vi "Copy FPGA SCTL.vi"(8 "error in (no error)":errorcluster, 11 "SCTL Name":string) -> (0 "error out":errorcluster)   [LabVIEW 2025, in "VI.lvclass"]
doc: "Copy a STCL from a template VI to be pasted into another VI."
uses:
  VI.lvclass
  VI.lvclass/VI.ctl
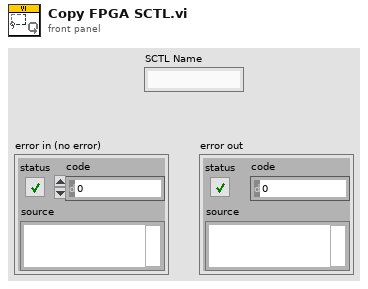
[diagram p1: front panel]
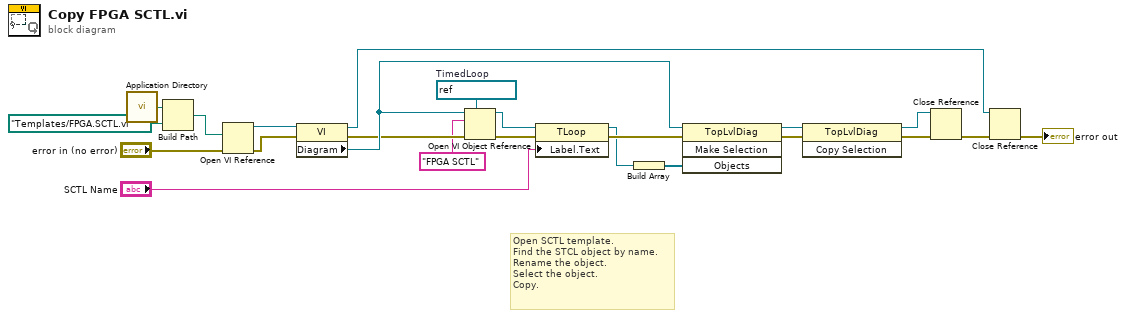
[diagram p0: block diagram]
diagram:
  w15 = refnum<vi> refnum  # TimedLoop
  # "Open SCTL template.\nFind the STCL object by name.\nRename the object.\nSelect the object.\nCopy."
  n1 = call <vilib>:"Application Directory.vi"() -> ("Application Directory"=w3:path)
  n2 = Build Path(base path=w3, name or relative path=path "Templates/FPGA.SCTL.vi" ("Application Directory")) -> (appended path=w1:path)
  n3 = Open VI Reference(vi path=w1, error in (no error)="error in (no error)") -> (vi reference=w9:refnum<vi>, error out=w13:errorcluster)  [unwired: 4 in]
  n4 = property class="VI"(reference=w9, error in=w13) -> (reference out=w20:refnum<vi>, error out=w17:errorcluster, "Diagram"=w18:refnum<vi>)
  n5 = Open VI Object Reference(7:w15, 8:w17, 10:"FPGA SCTL" ("name/order"), 11:w18) -> (0:w7:errorcluster, 3:w8:refnum<vi>)
  n6 = property class="TLoop"(reference=w8, error in=w7, "Label.Text"="SCTL Name") -> (reference out=w5:refnum<vi>, error out=w6:errorcluster)
  n7 = Build Array(w5) -> (w16:refnum<vi>[])
  n8 = invoke class="TopLvlDiag" method="Make Selection"(reference=w18, error in=w6, "Objects"=w16) -> (reference out=w10:refnum<vi>, error out=w11:errorcluster)  [unwired: 1 in, 2 out]
  n9 = invoke class="TopLvlDiag" method="Copy Selection"(reference=w10, error in=w11) -> (reference out=w22:refnum<vi>, error out=w21:errorcluster)  [unwired: 1 in, 1 out]
  n10 = Close Reference(reference=w22, error in (no error)=w21) -> (error out=w23:errorcluster)
  n11 = Close Reference(reference=w20, error in (no error)=w23) -> (error out=→"error out":errorcluster)
